vi "Flatten To String.vi"(8 "error in (no error)":errorcluster, 10 "Record":refnum<class "Record.lvclass">, 11 "Serializer in":refnum<class "Serializer.lvclass">) -> (0 "error out":errorcluster, 2 "Flattened String":string, 3 "Serializer out":refnum<class "Serializer.lvclass">)   [LabVIEW 2017, in "Error Log.lvlib" / "Serializer.lvclass"]
uses:
  Serializer.lvclass
  Record/Record.lvclass
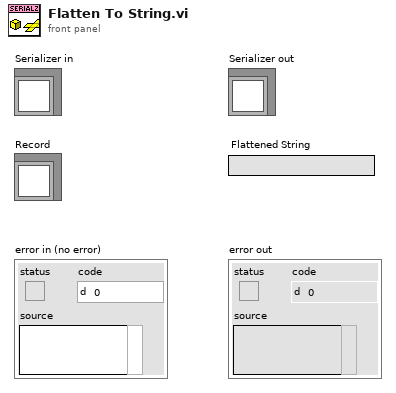
[diagram p1: front panel]
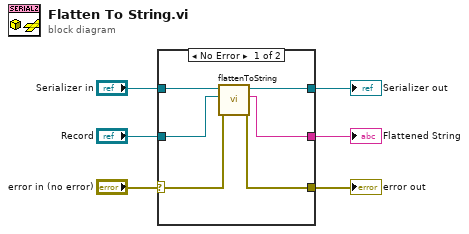
[diagram p0: block diagram]
diagram:
  n1 = case shown="No Error" "error in (no error)" {
    selector: "error in (no error)" -> [w10 w14]
    tunnel: [w9 w14] -> w5
    tunnel: [w11 w13] -> w3
    tunnel: "Serializer in" -> [w12 w13]
    tunnel: "Record" -> [w8 _]
    tunnel: [w7 _] -> w1
    frame No Error {
      n2 = call-dynamic "flattenToString.vi"("error in (no error)"=w10, "Record"=w8, "Serializer in"=w12) -> ("error out"=w9:errorcluster, "Flattened String"=w7:string, "Serializer out"=w11:refnum<class "Serializer.lvclass">)  [unwired: 6 in]
    }
    frame Error {
    }
  }
  "error out" <- w5
  "Serializer out" <- w3
  "Flattened String" <- w1
